vi "Change Cell Padding.vi"(0 "String":string, 7 "String (Char U16 [ ])":u16[](array[numeric]), 11 "error in (no error)":errorcluster, 12 "Font":refnum<k24>, 13 "Type and run direction":T1=enum."ASCII") -> (8 "Change cell padding?":bool, 10 "Size":sgl, 15 "error out duplicate":errorcluster)   [LabVIEW 2019]
doc: "Developed by Jean-Marc Simard\nCopyright © 2012, Exaprom Inc.\nAll rights reserved.\nLicense: BSD\n\nWith iTextSharp 4.1.6 (http://itextsharp.sourceforge.net)\nunder Mozilla Public License Version 1.1\n(http://www.mozilla.org/MPL/MPL-1.1.html)"
uses:
  <userlib>/Exaprom PDF/Controls/Text Controls/Unicode/Type and run direction.ctl
  C:/Program Files/National Instruments/LabVIEW 2019/user.lib/Exaprom PDF/DLL/itextsharp.dll
  DLL/itextsharp.dll
  <userlib>/Exaprom PDF/VIs/Low level/General/Binary Search 1D Array.llb/Binary Search 1D Array (U16).vi
  <vilib>/regexp/Match Regular Expression.xnode
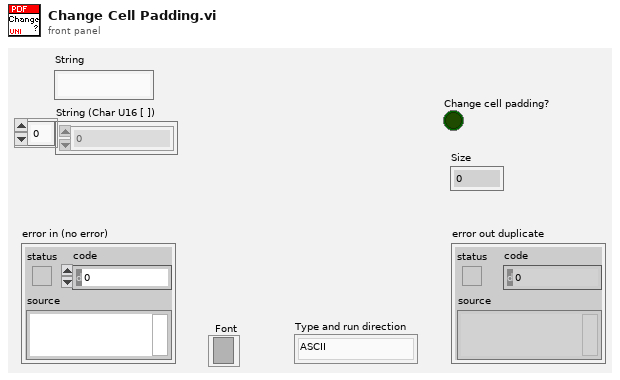
[diagram p1: front panel]
types:
  T1 = typedef "Type and run direction.ctl" = enum16{"Select", "ASCII", "UTF-16", "UTF-16 (default)", "UTF-16 (LTR)", "UTF-16 (RTL)"}
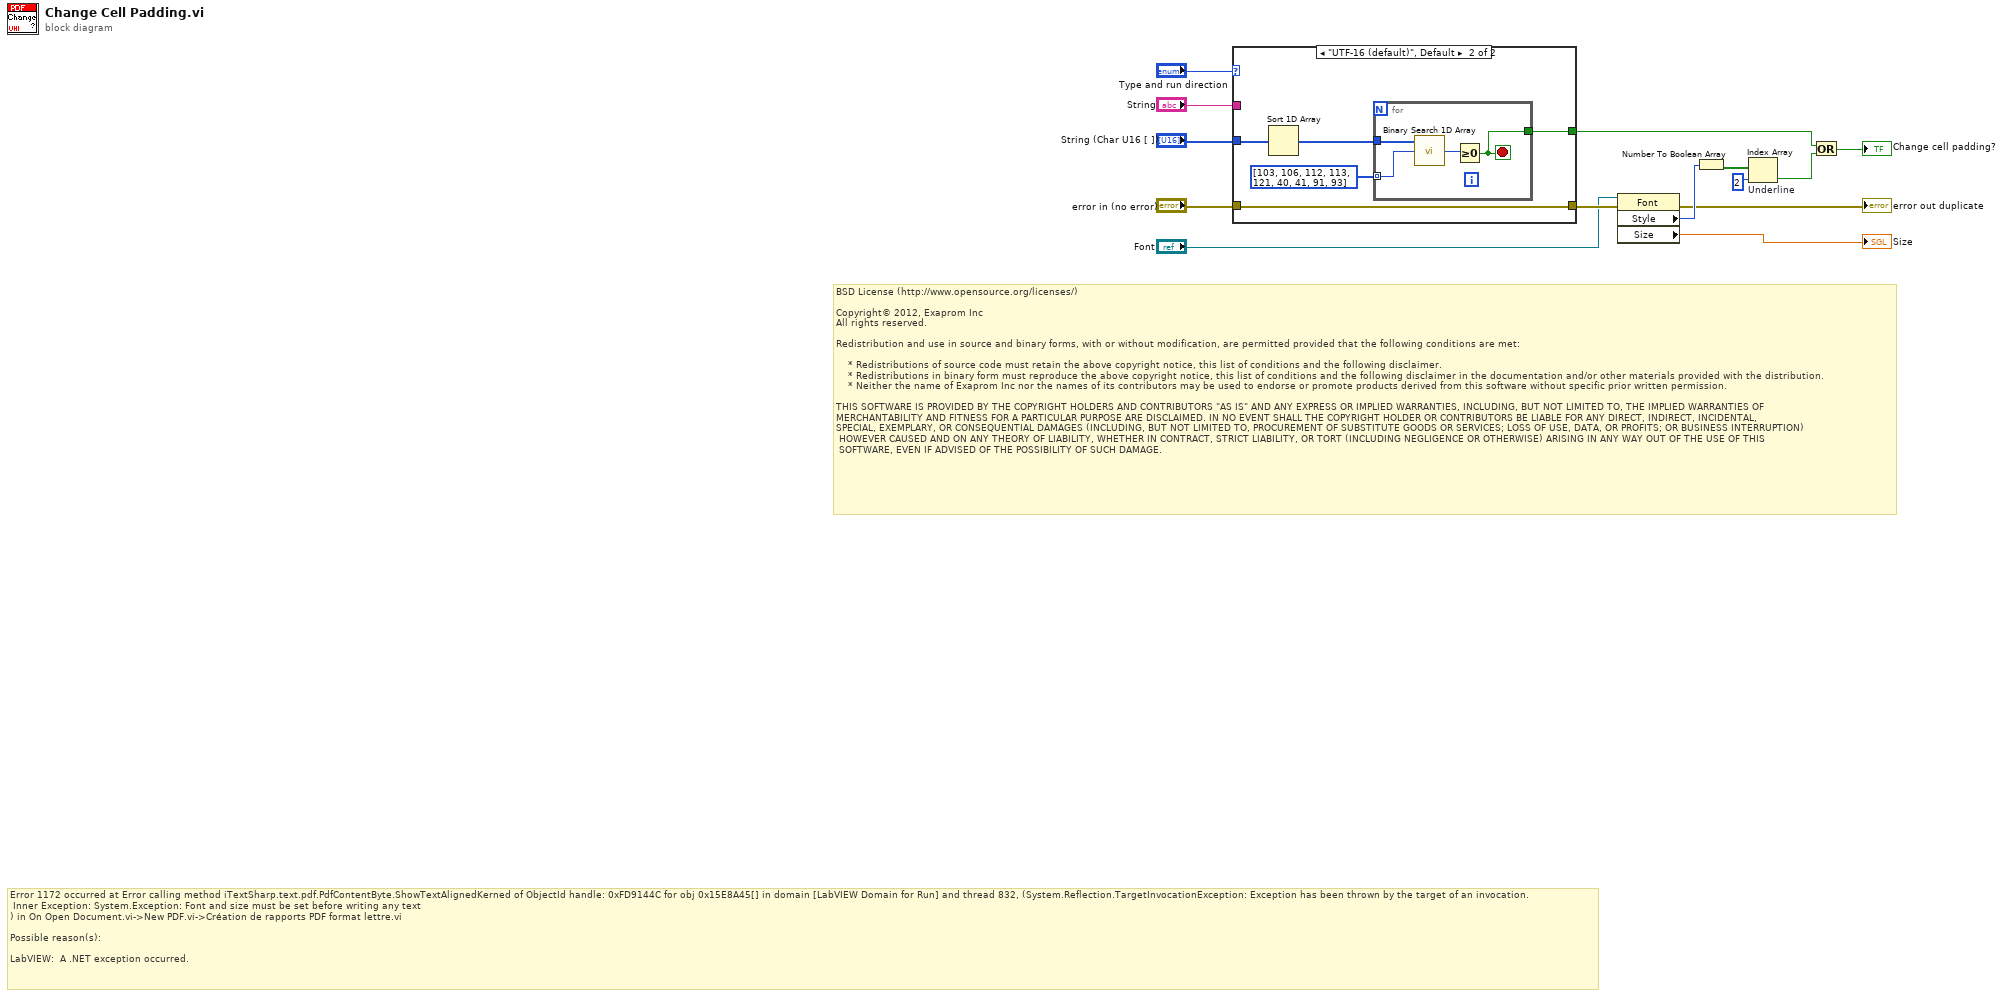
[diagram p0: block diagram]
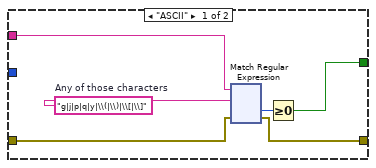
[diagram p2: hidden frame]
diagram:
  # "Error 1172 occurred at Error calling method iTextSharp.text.pdf.PdfContentByte.ShowTextAlignedKerned of ObjectId handle: 0xFD9144C for obj 0x15E8A45[] in domain [LabVIEW Domain for Run] and thread 832, (System.Reflection.TargetInvocationException: Exception has been thrown by the target of an invocation.\n\tInner Exception: System.Exception: Font and size must be set before writing any text\n) in On Open Document.vi->New PDF.vi->Création de rapports PDF format lettre.vi\n\nPossible reason(s):\n\nLabVIEW:  A .NET exception occurred."
  # "BSD License (http://www.opensource.org/licenses/)\n\nCopyright© 2012, Exaprom Inc\nAll rights reserved.\n\nRedistribution and use in source and binary forms, with or without modification, are permitted provided that the following conditions are met:\n\n    * Redistributions of source code must retain the above copyright notice, this list of conditions and the following disclaimer.\n    * Redistributions in binary form must reproduce the above copyright notice, this list of conditions and the following disclaimer in the documentation and/or other materials provided with the distribution.\n    * Neither the name of Exaprom Inc nor the names of its contributors may be used to endorse or promote products derived from this software without specific prior written permission.\n\nTHIS SOFTWARE IS PROVIDED BY THE COPYRIGHT HOLDERS AND CONTRIBUTORS \"AS IS\" AND ANY EXPRESS OR IMPLIED WARRANTIES, INCLUDING, BUT NOT LIMITED TO, THE IMPLIED WARRANTIES OF \nMERCHANTABILITY AND FITNESS FOR A PARTICULAR PURPOSE ARE DISCLAIMED. IN NO EVENT SHALL THE COPYRIGHT HOLDER OR CONTRIBUTORS BE LIABLE FOR ANY DIRECT, INDIRECT, INCIDENTAL,\nSPECIAL, EXEMPLARY, OR CONSEQUENTIAL DAMAGES (INCLUDING, BUT NOT LIMITED TO, PROCUREMENT OF SUBSTITUTE GOODS OR SERVICES; LOSS OF USE, DATA, OR PROFITS; OR BUSINESS INTERRUPTION)\n HOWEVER CAUSED AND ON ANY THEORY OF LIABILITY, WHETHER IN CONTRACT, STRICT LIABILITY, OR TORT (INCLUDING NEGLIGENCE OR OTHERWISE) ARISING IN ANY WAY OUT OF THE USE OF THIS\n SOFTWARE, EVEN IF ADVISED OF THE POSSIBILITY OF SUCH DAMAGE."
  n1 = case shown="\"UTF-16 (default)\", Default" "Type and run direction" {
    tunnel: "String (Char U16 [ ])" -> [_ w139]
    tunnel: [w17 w137] -> w5
    tunnel: "String" -> [w18 _]
    tunnel: "error in (no error)" -> [w16 w136]
    tunnel: [w15 w136] -> w7
    frame "ASCII" {
      w20 = "g|j|p|q|y|\\(|\\)|\\[|\\]"  # Any of those characters
      n2 = xnode "Match Regular Expression"("input string"=w18, "regular expression"=w20, "error in"=w16) -> ("offset past match"=w19:i32, "error out"=w15:errorcluster)  [unwired: 1 in, 5 out]
      n3 = Greater Or Equal To 0?(x=w19) -> (x >= 0?=w17:bool)
    }
    frame "UTF-16 (default)", Default {
      n4 = Sort 1D Array(array=w139) -> (sorted array=w138:u16[])
      n5 = for {
        tunnel: w138 -> [w143]
        tunnel: u16[] [103, 106, 112, 113, 121, 40, 41, 91, 93] ("Any of those (Char U16 [ ])") -> [w142] mode=indexing
        tunnel: [w140] -> w137
        stop <- w140 stop-if-true
        n6 = call-poly <userlib>:"Binary Search 1D Array.vi"("element"=w142, "1D array"=w143) -> ("index"=w141:i32)  [unwired: 1 in]
        n7 = Greater Or Equal To 0?(x=w141) -> (x >= 0?=w140:bool)
      }
    }
  }
  n8 = property class="Font"(reference="Font", error in=w7) -> (error out=→"error out duplicate":errorcluster, "Style"=w13:i32, "Size"=→"Size":sgl)  [unwired: 1 out]
  n9 = Number To Boolean Array(number=w13) -> (Boolean array=w12:bool[])
  n10 = Index Array "Underline"(array=w12, index=2) -> (element=w4:bool)
  n11 = Or(x=w5, y=w4) -> (x .or. y?=→"Change cell padding?":bool)
